vi "Global.vi"() -> ()   [LabVIEW 2013]
panel:
  in  "set angle down":bool
  in  "set angle up":bool
  in  "Rightpositionsetpoint":dbl
  in  "Leftpositionsetpoint":dbl
  in  "ToggleAngle?":bool
  in  "Launch?":bool
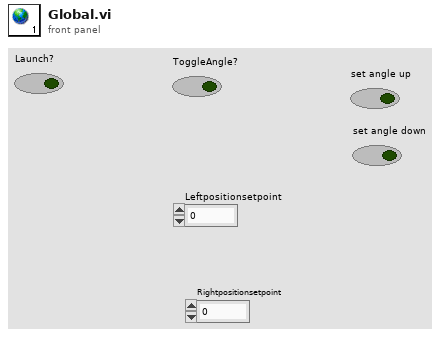
[diagram p1: front panel]
diagram:
